vi "peak_detection_2d.vi"(10 "2d spectra cluster":T1(array[cluster])) -> ()   [LabVIEW 2012]
uses:
  <vilib>/Analysis/baseanly.llb/Mean (DBL).vi
  <vilib>/measure/NI_MAPro.lvlib
  <vilib>/Analysis/NI_AALBase.lvlib
panel:
  out "Waveform Graph":T1(graph) caption="Combined Spectra"
  in  "Select Frequency Step":i32=1 min=1 max=5
  in  "Stop":bool
  out "Amplitude":dbl[](array[numeric]) format="%.3p"
  out "Frequency":dbl[](array[numeric]) format="%.6p"
  out "Average Cor":cluster{"Array":dbl[], "magnitude":dbl[]}[](graph)
  in  "Threshold Value":dbl=10.0
  out "Peaks Found":i32
  in  "Minimum Peak Width":i32=5 min=3
  # "Detection Settings"
  # "Detected Peaks"
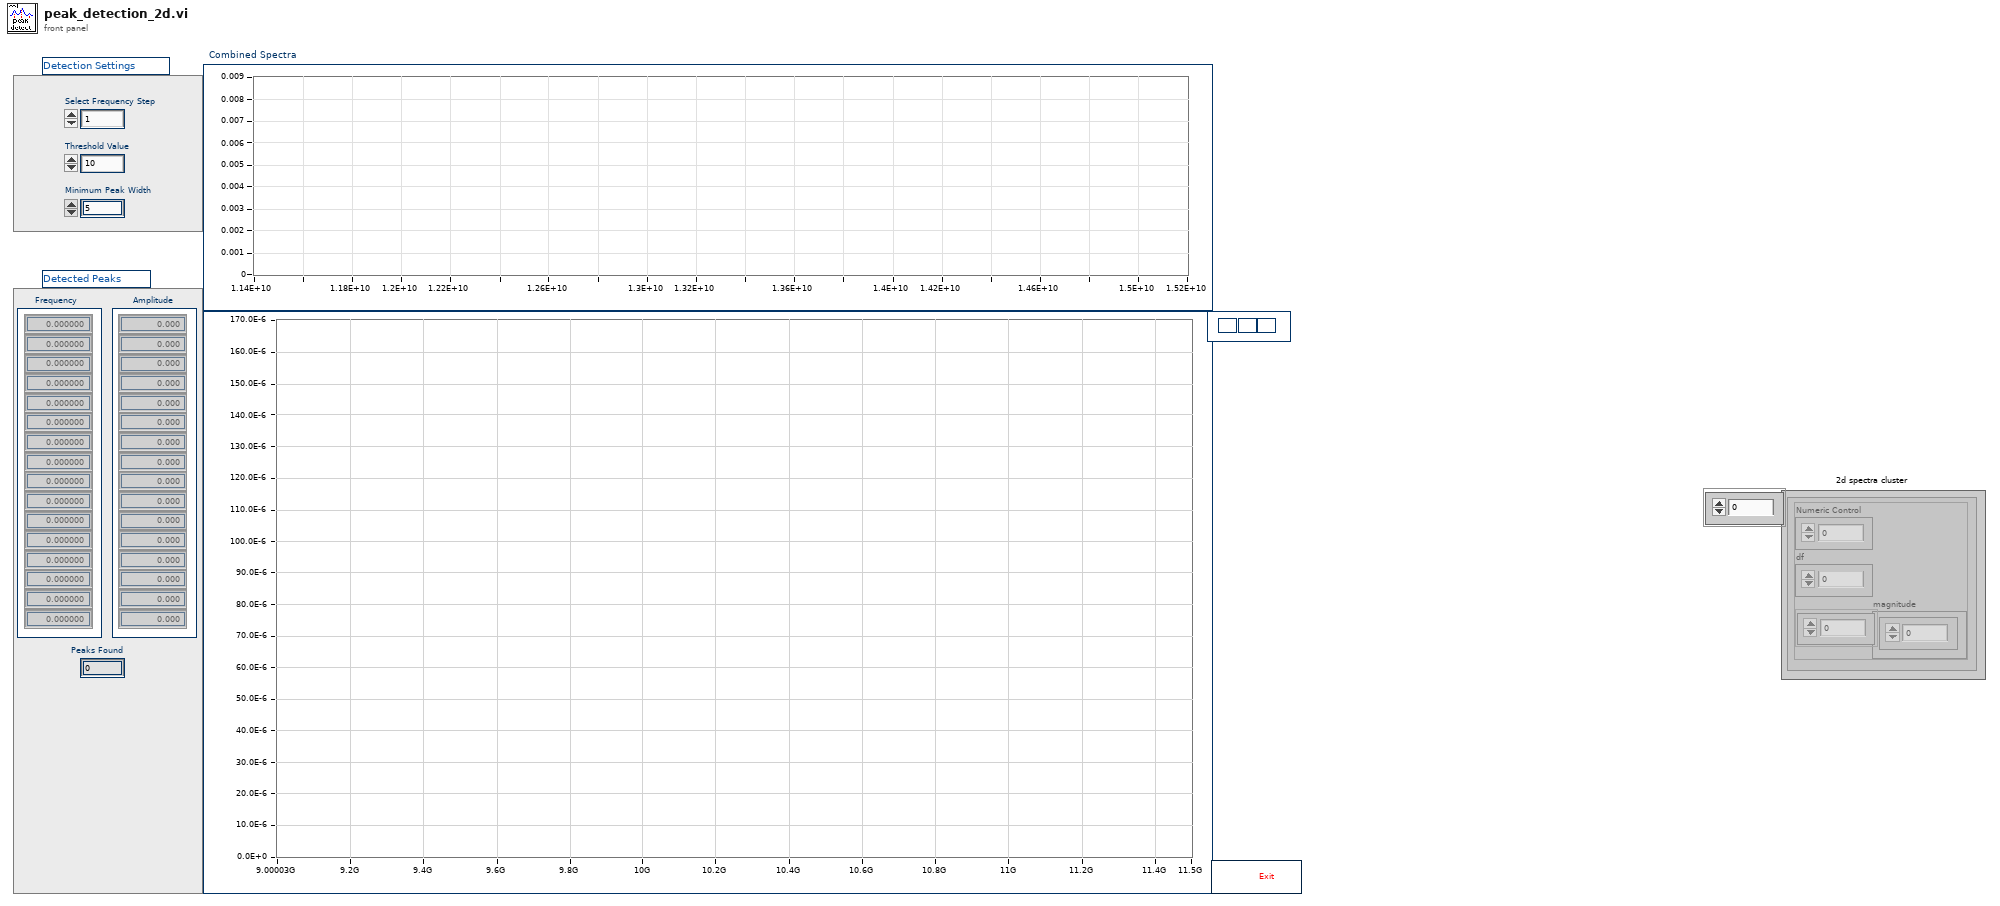
[diagram p1: front panel]
types:
  T1 = cluster{"Numeric Control":dbl, "df":dbl, "magnitude":dbl[]}[]
  T2 = cluster{"Numeric Control":dbl, "df":dbl, "magnitude":dbl[]}
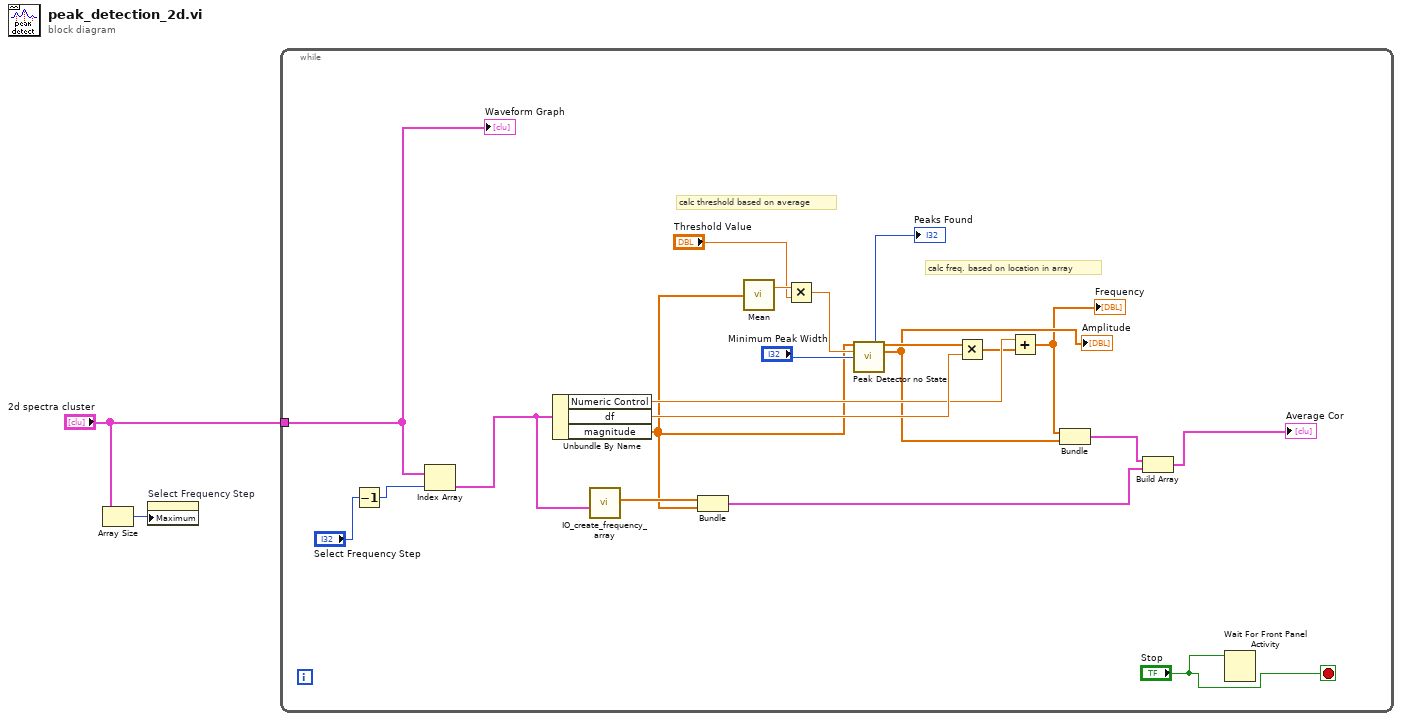
[diagram p0: block diagram]
diagram:
  n1 = Array Size(array="2d spectra cluster") -> (size(s)=w1:i32)
  n2 = property on="Select Frequency Step" class="DigNum (strict)"("Maximum"=w1) -> ()  [unwired: 2 in, 2 out]
  n3 = while {
    tunnel: "2d spectra cluster" -> [w3]
    stop <- "Stop" stop-if-true
    # "calc freq. based on location in array"
    # "calc threshold based on average"
    n4 = Decrement(x="Select Frequency Step") -> (x-1=w8:i32)
    n5 = Index Array(array=w3, index=w8) -> (element=w10:T2)
    n6 = Unbundle By Name(w10) -> ("Numeric Control"=w17:dbl, "df"=w18:dbl, "magnitude"=w13:dbl[])
    n7 = call "IO_create_frequency_array.vi"("cor"=w10) -> ("Array"=w14:dbl[])  [unwired: 9 in, 1 out]
    n8 = Bundle("Array"=w14, "magnitude"=w13) -> (w11:cluster{"Array":dbl[], "magnitude":dbl[]})  [unwired: 1 in]
    n9 = call-poly <vilib>:"Mean.vi"("X"=w13) -> ("mean"=w21:dbl)  [unwired: 1 out]
    n10 = Multiply(x=w21, y="Threshold Value") -> (x*y=w15:dbl)
    n11 = call <vilib>:"Peak Detector no State.vi"("X"=w13, "threshold"=w15, "width"="Minimum Peak Width") -> ("# found"=→"Peaks Found":i32, "Locations"=w19:dbl[], "Amplitudes"=w5:dbl[])  [unwired: 5 in, 5 out]
    "Amplitude" <- w5
    n12 = Multiply(x=w19, y=w18) -> (x*y=w16:dbl[])
    n13 = Add(x=w17, y=w16) -> (x+y=w4:dbl[])
    "Frequency" <- w4
    n14 = Bundle(w4, "Amplitudes"=w5) -> (w12:cluster{dbl[], "Amplitudes":dbl[]})  [unwired: 1 in]
    n15 = Build Array(w12, w11) -> (→"Average Cor":cluster{"Array":dbl[], "magnitude":dbl[]}[])
    n16 = Wait For Front Panel Activity(3:"Stop") -> ()  [unwired: 2 in, 1 out]
    "Waveform Graph" <- w3
  }
